vi "UFO.vi"(11 "VI Ref":refnum<vi>) -> ()   [LabVIEW 2019]
doc: "UFO disaster. A UFO will spawn at a random location on the top edge of the screen, then slowly move down the screen destroying any objects in its path."
uses:
  _SubVIs/UFO State Enum.ctl
  _SubVIs/Slave Window Command Message.ctl
  _SubVIs/Slave Window Command.ctl
  _Sound/Music Player Command Message.ctl
  _Sound/Music Player Command.ctl
  _2D/Point.ctl
  <vilib>/Utility/miscctls.llb/LVRectTypeDef.ctl
  <vilib>/numeric/Random Number (Range).vi
  <vilib>/numeric/Random Number (Range) I64.vi
  <vilib>/numeric/sub_Random U32.vi
  _Window/Window.lvlib
  _Sound/Sound.lvlib
  _2D/2D.lvlib
panel:
  out "Attack":u16(ring)
  out "UFO":u16(ring)
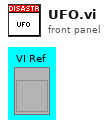
[diagram p1: front panel]
types:
  T1 = enum32{"Invalid", "Standard", "Closed", "Hidden", "Minimized", "Maximized"}
  T2 = typedef "LVRectTypeDef.ctl" = cluster{"Left":i16, "Top":i16, "Right":i16, "Bottom":i16}
  T3 = typedef "2D.lvlib/Point.ctl" = cluster{"X":i16, "Y":i16}
  T4 = typedef "UFO State Enum.ctl" = enum16{"Init", "Init Window", "Play Music", "Fade In Window", "Update Time", "Update Window Position", "Check Window Over BD", "Object Collision Detection", "Update Graphic", "Fade Out Window", "Close Window"}
  T5 = typedef "Sound.lvlib/Music Player Command Message.ctl" = cluster{"Command":T6, "Data":variant}
  T6 = typedef "Sound.lvlib/Music Player Command.ctl" = enum16{"Enable", "Play", "Play Random", "Stop", "Shutdown"}
  T7 = typedef "Slave Window Command Message.ctl" = cluster{"Command":T8, "Data":variant}
  T8 = typedef "Slave Window Command.ctl" = enum16{"Open", "Set Bounds", "Set Opacity", "Close", "Frame"}
  T9 = cluster{"BDWin.NativeWindow":u64, "vi reference":refnum<vi>}[]
  T10 = typedef "LVPointTypeDef.ctl" = cluster{"Horizontal":i16, "Vertical":i16}
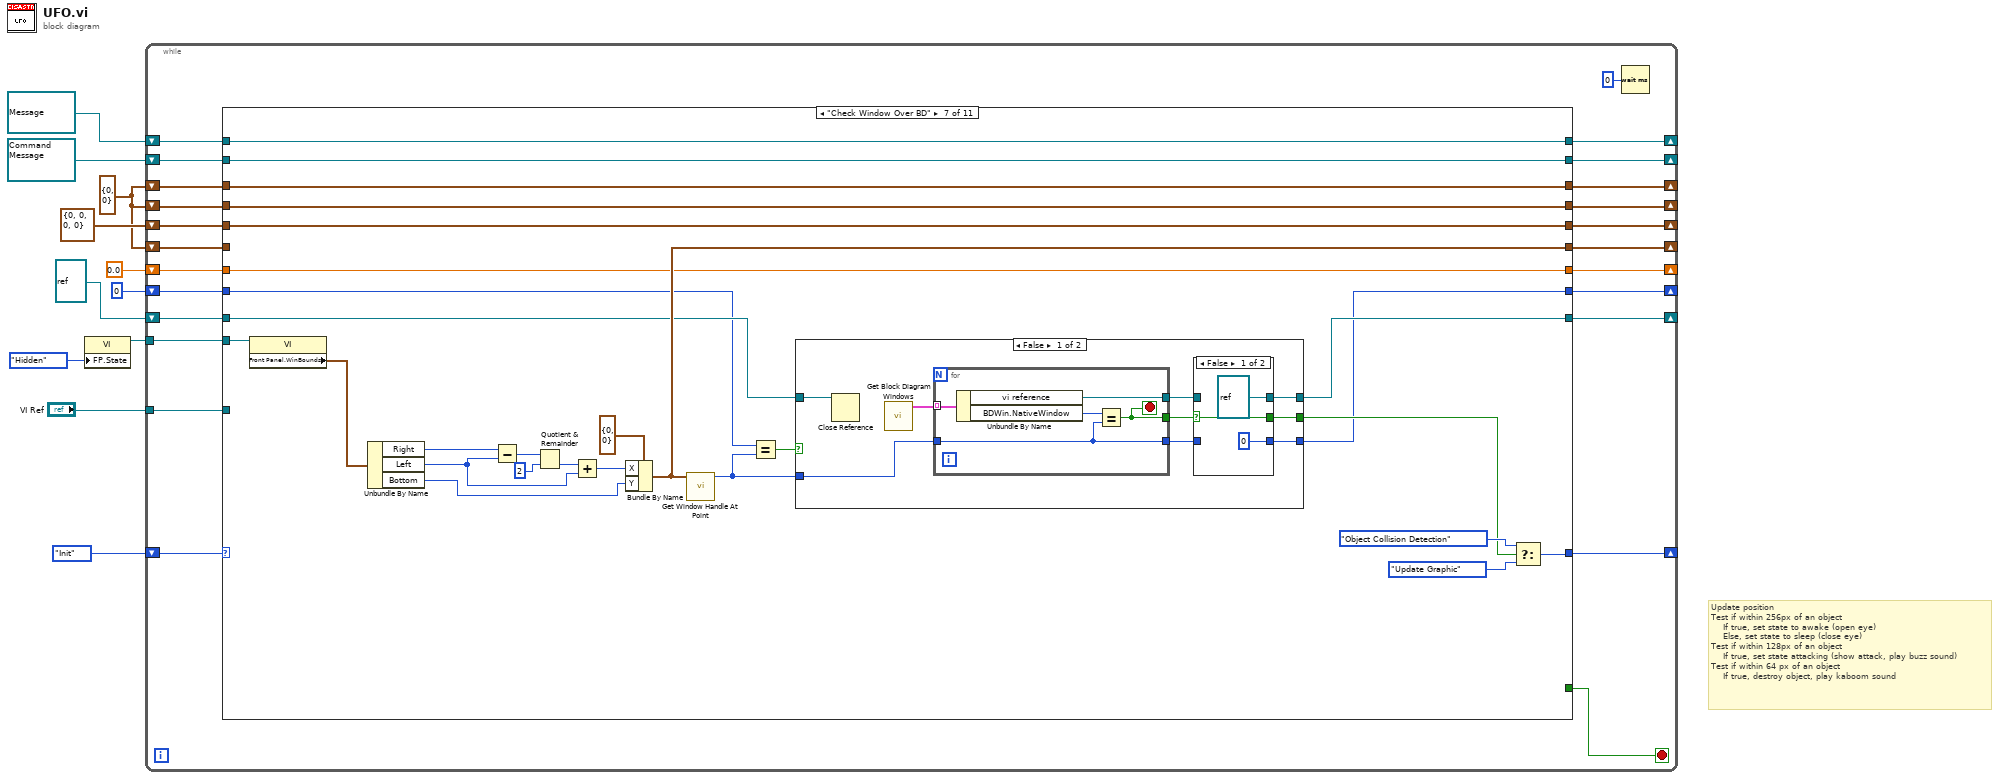
[diagram p0: block diagram]
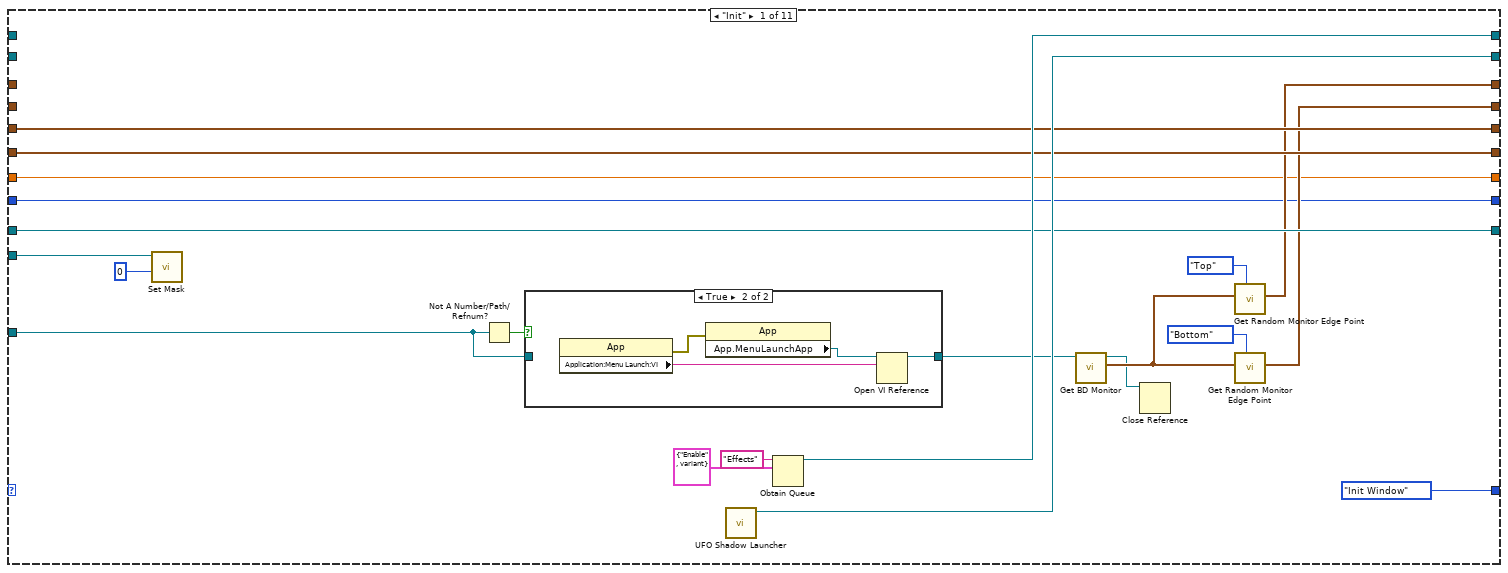
[diagram p2: hidden frame]
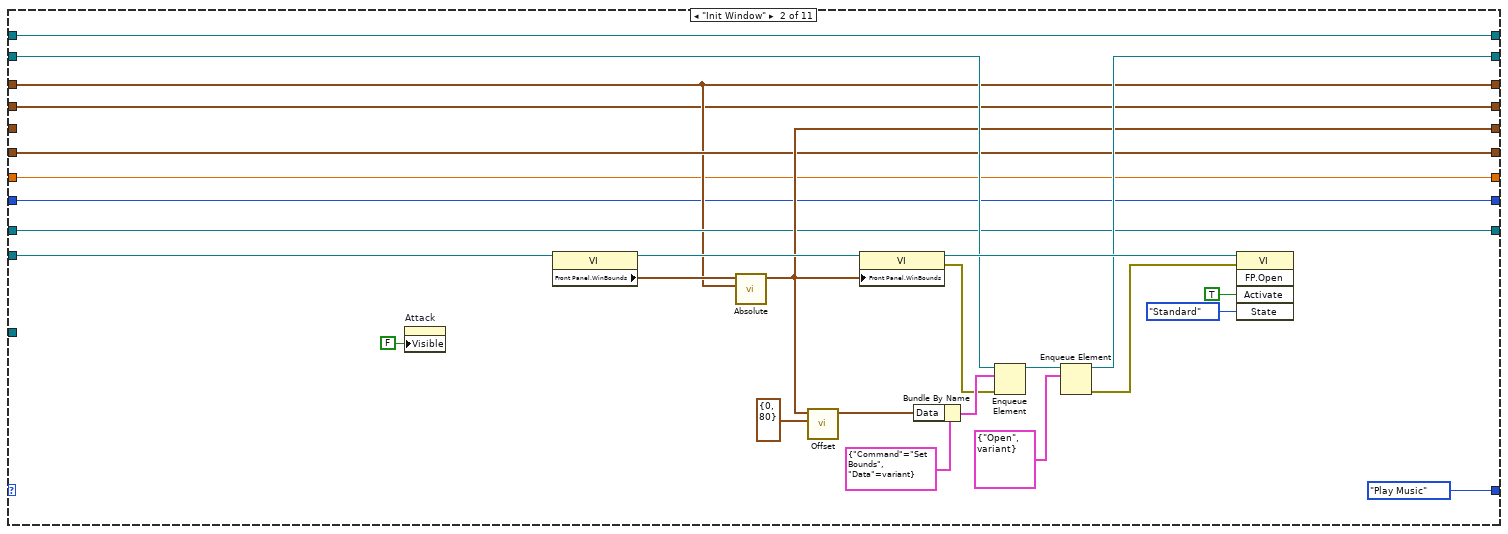
[diagram p4: hidden frame]
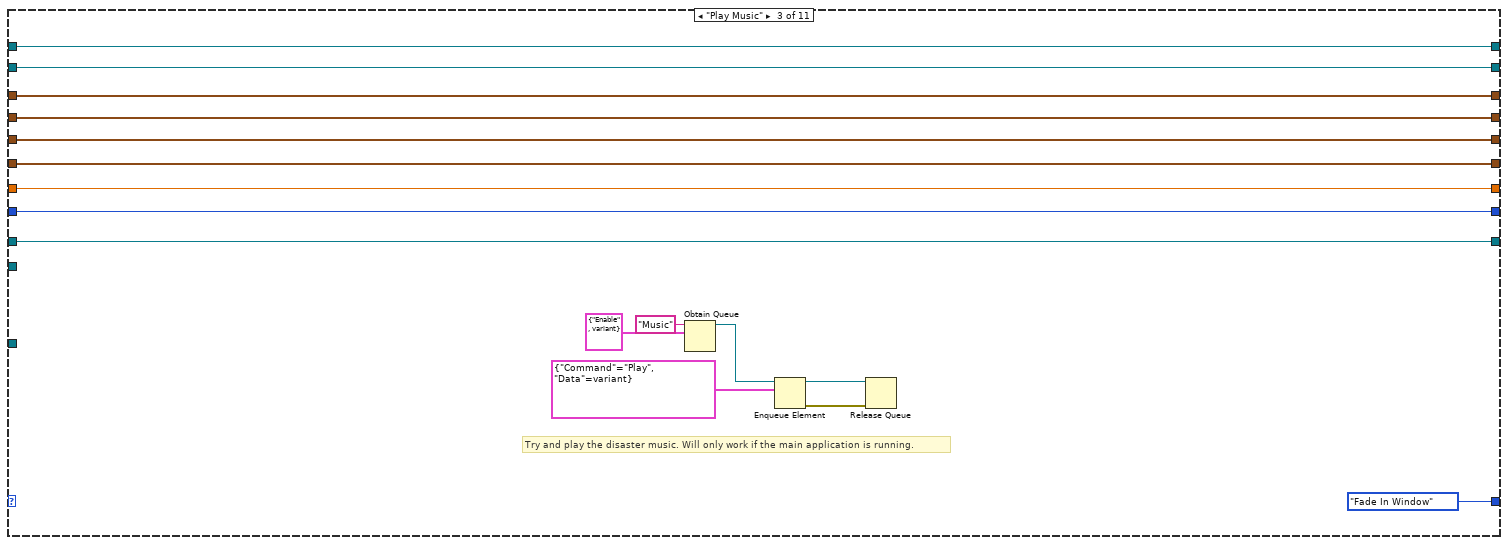
[diagram p5: hidden frame]
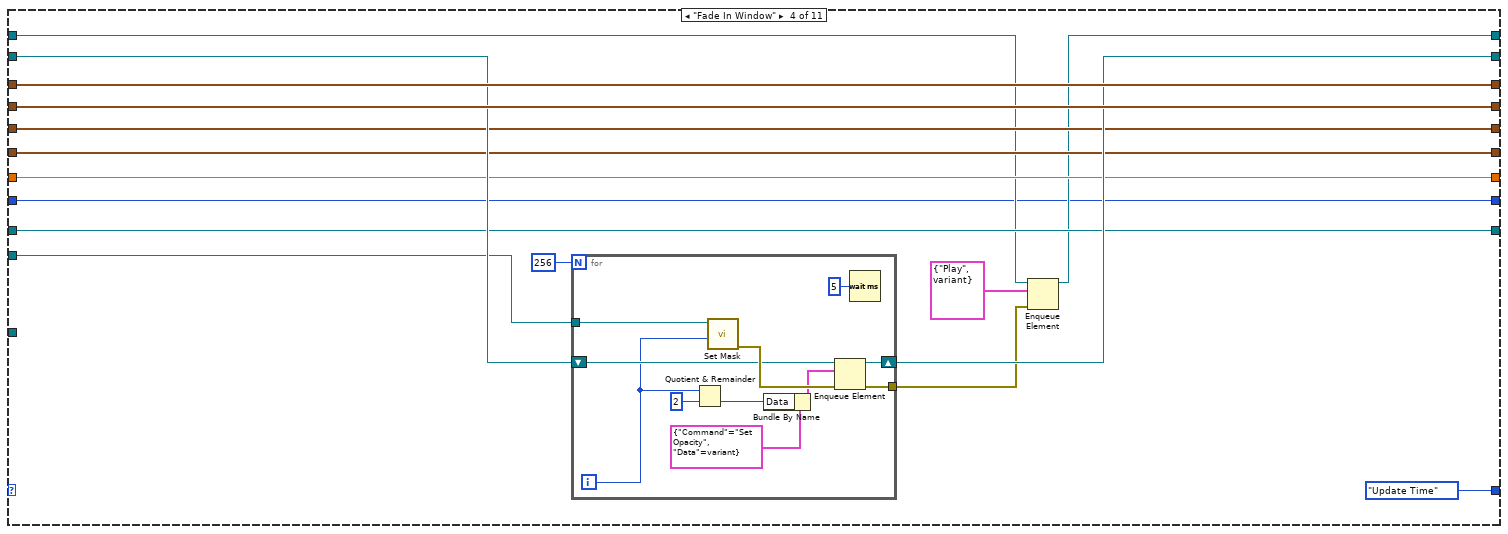
[diagram p6: hidden frame]
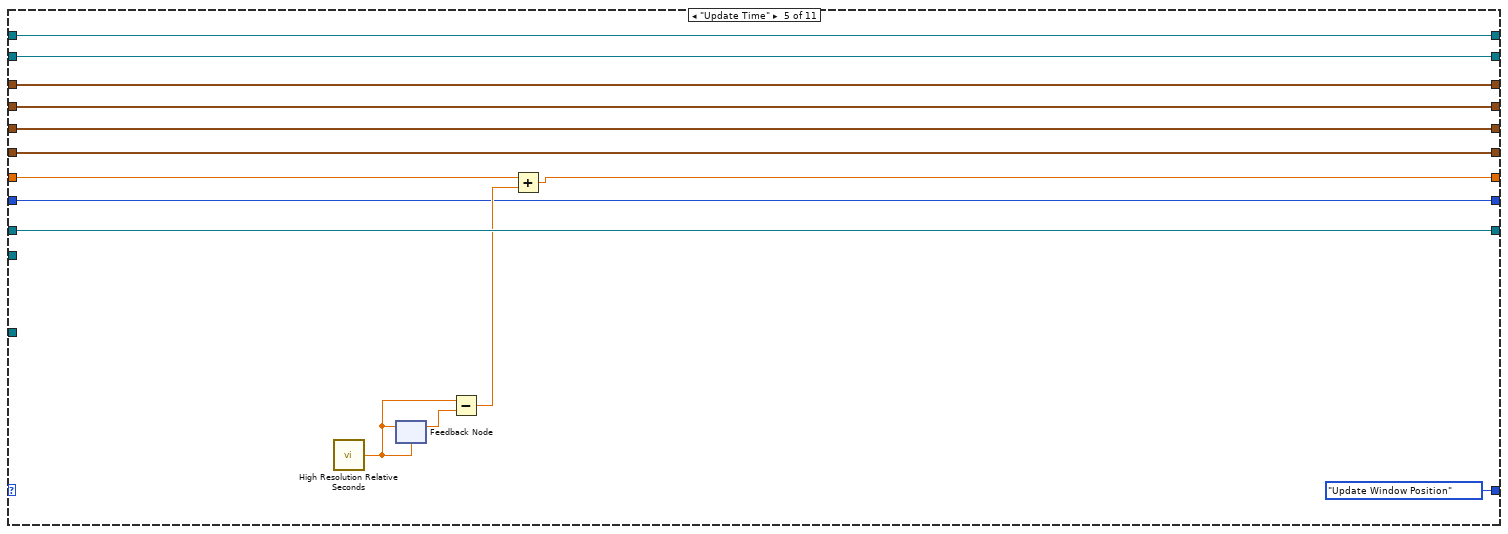
[diagram p7: hidden frame]
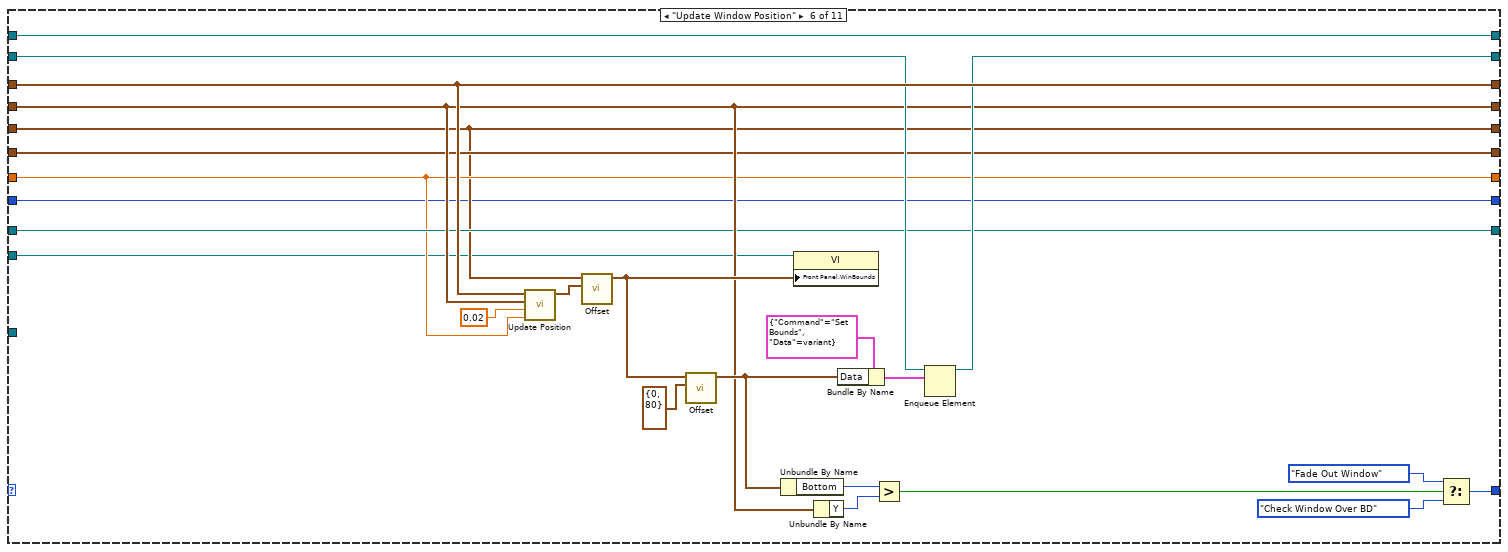
[diagram p8: hidden frame]
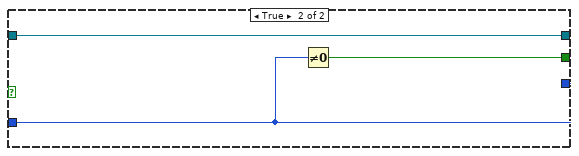
[diagram p10: hidden frame]
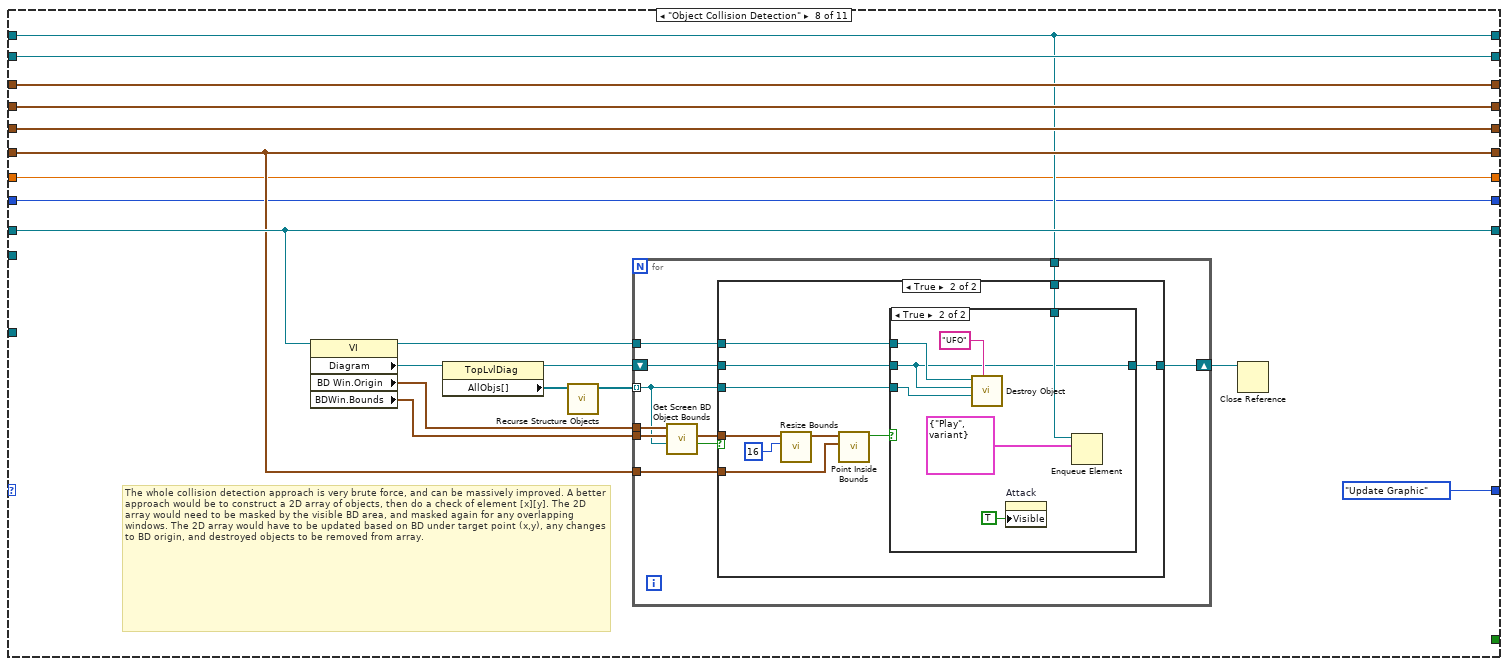
[diagram p11: hidden frame]
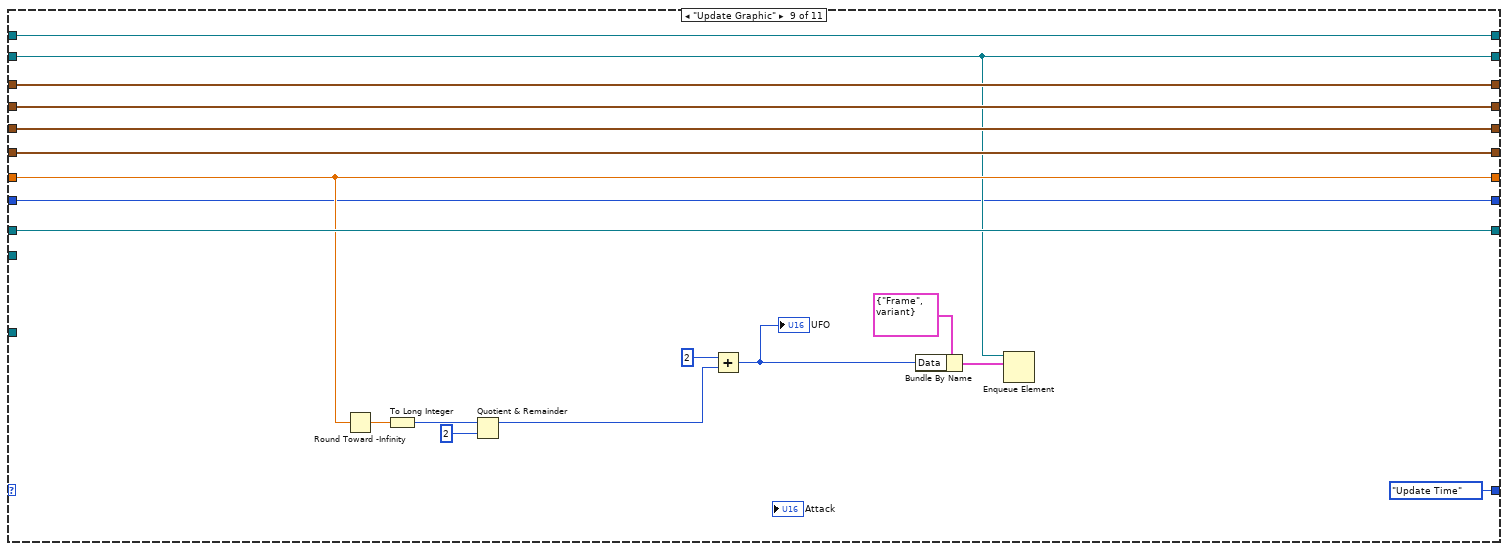
[diagram p14: hidden frame]
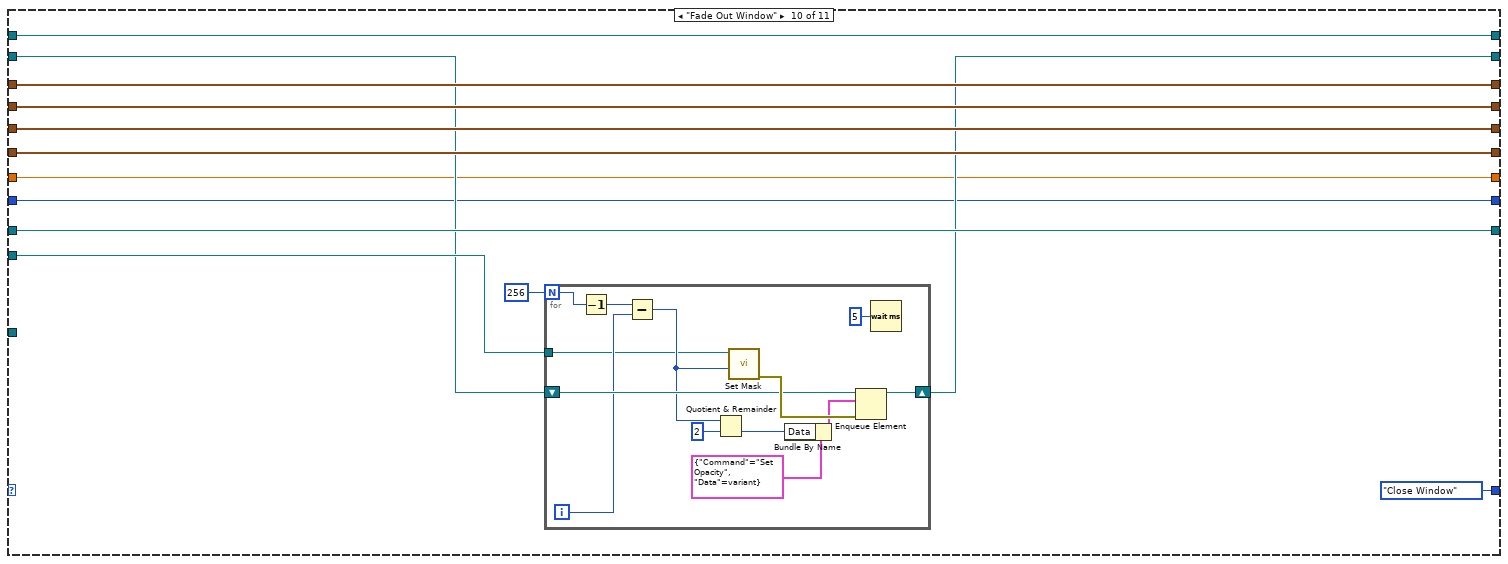
[diagram p15: hidden frame]
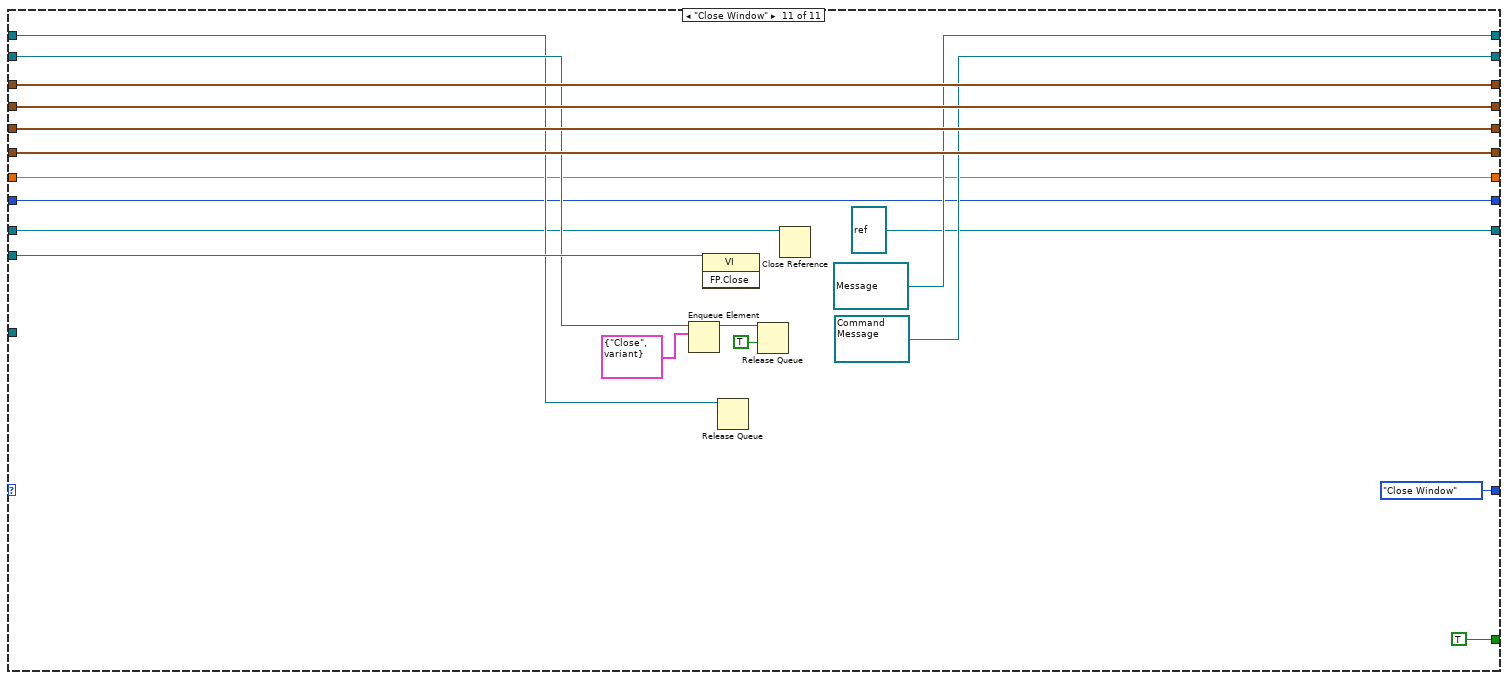
[diagram p16: hidden frame]
diagram:
  w6 = T3 {"X"=0, "Y"=0} ("Point")
  # "Update position\nTest if within 256px of an object\n    If true, set state to awake (open eye)\n    Else, set state to sleep (close eye)\nTest if within 128px of an object\n    If true, set state attacking (show attack, play buzz sound)\nTest if within 64 px of an object\n    If true, destroy object, play kaboom sound"
  n1 = property class="VI"("FP.State"=T1."Hidden" ("Front Panel Window:State")) -> (reference out=w2:refnum<vi>)  [unwired: 2 in, 1 out]
  n2 = while {
    shift-right: [w31] -> _
    shift-left: UFO_State_Enum."Init" -> [w35]
    tunnel: w2 -> [w30]
    shift-right: [w33] -> _
    shift-left: refnum<queue> refnum ("Command Queue") -> [w29]
    shift-right: [w32] -> _
    shift-left: refnum<queue> refnum ("queue out") -> [w28]
    shift-right: [w27] -> _
    shift-left: w6 -> [w25]
    shift-right: [w26] -> _
    shift-left: w6 -> [w24]
    shift-right: [w23] -> _
    shift-left: T2 {"Left"=0, "Top"=0, "Right"=0, "Bottom"=0} ("Bounds Out") -> [w22]
    shift-right: [w21] -> _
    shift-left: refnum<vi> refnum ("vi reference") -> [w18]
    shift-right: [w20] -> _
    shift-left: w6 -> [w19]
    tunnel: "VI Ref" -> [w34]
    shift-right: [w15] -> _
    shift-left: 0.0 -> [w16]
    shift-right: [w13] -> _
    shift-left: 0 ("hWnd") -> [w12]
    stop <- w17 stop-if-true
    n3 = case shown="\"Check Window Over BD\"" w35 {
      tunnel: w34 -> [w54 _ _ _ _ _ _ _ _ _ _]
      tunnel: [w52 w69 w96 w116 w144 w157 w195 w236 w274 w288 refnum<queue> refnum ("Command Queue")] -> w33
      tunnel: [w51 w70 w97 w107 w143 w168 w194 w222 w283 w296 refnum<queue> refnum ("queue out")] -> w32
      tunnel: [UFO_State_Enum."Init Window" UFO_State_Enum."Play Music" UFO_State_Enum."Fade In Window" UFO_State_Enum."Update Time" UFO_State_Enum."Update Window Position" w152 w180 UFO_State_Enum."Update Graphic" UFO_State_Enum."Update Time" UFO_State_Enum."Close Window" UFO_State_Enum."Close Window"] -> w31
      tunnel: w30 -> [w38 w74 _ w110 _ w146 w182 _ _ w289 w320]
      tunnel: w29 -> [_ w72 w96 w115 w144 w156 w195 w236 w274 w287 w319]
      tunnel: w28 -> [_ w70 w97 w106 w143 w168 w194 w222 w283 w296 w318]
      tunnel: [w42 w65 w95 w118 w142 w158 w193 w235 w282 w295 w327] -> w27
      tunnel: [w41 w64 w94 w117 w141 w151 w192 w234 w281 w294 w326] -> w26
      tunnel: w25 -> [_ w65 w95 w118 w142 w158 w193 w235 w282 w295 w327]
      tunnel: w24 -> [_ w64 w94 w117 w141 w151 w192 w234 w281 w294 w326]
      tunnel: [w49 w68 w92 w113 w140 w147 w191 w233 w280 w293 w325] -> w23
      tunnel: w22 -> [w49 _ w92 w113 w140 w147 w191 w233 w280 w293 w325]
      tunnel: [w47 w66 w90 w111 w139 w149 w174 w227 w279 w292 refnum<vi> refnum ("vi reference")] -> w21
      tunnel: [w48 w67 w91 w112 w138 w150 w177 w226 w278 w291 w324] -> w20
      tunnel: w19 -> [w48 w67 w91 w112 w138 w150 _ w226 w278 w291 w324]
      tunnel: w18 -> [w47 w66 w90 w111 w139 w149 w173 w227 w279 w292 w311]
      tunnel: [_ _ _ _ _ _ _ _ _ _ TRUE] -> w17
      tunnel: w16 -> [w40 w63 w89 w109 w135 w148 w176 w221 w275 w285 w313]
      tunnel: [w40 w63 w89 w109 w132 w148 w176 w221 w275 w285 w313] -> w15
      tunnel: [w37 w62 w88 w104 w131 w145 w172 w220 w266 w284 w312] -> w13
      tunnel: w12 -> [w37 w62 w88 w104 w131 w145 w171 w220 w266 w284 w312]
      frame "Init" {
        n4 = call "Set Mask.vi"("Alpha (255)"=0, "VI Ref In"=w38) -> ()  [unwired: 8 in, 2 out]
        n5 = Not A Number/Path/Refnum?(number/path/refnum=w54) -> (NaN/Path/Refnum?=w53:bool)
        n6 = case shown="True" w53 {
          tunnel: w54 -> [w57 _]
          tunnel: [w57 w60] -> w43
          frame False {
          }
          frame True {
            n7 = property class="App"() -> (error out=w59:errorcluster, "Application:Menu Launch:VI"=w61:string)  [unwired: 2 in, 1 out]
            n8 = property class="App"(error in=w59) -> ("App.MenuLaunchApp"=w58:refnum<vi>)  [unwired: 1 in, 2 out]
            n9 = Open VI Reference(application reference (local)=w58, vi path=w61) -> (vi reference=w60:refnum<vi>)  [unwired: 4 in, 1 out]
          }
        }
        n10 = call "UFO Shadow Launcher.vi"() -> ("Command Queue"=w52:refnum<queue>)  [unwired: 10 in, 1 out]
        n11 = Obtain Queue(name (unnamed)="Effects", element data type=T5 {"Command"=enum."Enable", "Data"=variant} ("Message")) -> (queue out=w51:refnum<queue>)  [unwired: 3 in, 2 out]
        n12 = call "Get BD Monitor.vi"("VI Ref In"=w43) -> ("Monitor Bounds"=w46:T2, "VI Ref Out"=w36:refnum<vi>)  [unwired: 8 in, 1 out]
        n13 = Close Reference(reference=w36) -> ()  [unwired: 1 in, 1 out]
        n14 = call "Get Random Monitor Edge Point.vi"("Edge"=enum16{"Left", "Top", "Right", "Bottom"}."Top", "Monitor Bounds"=w46) -> ("Point"=w42:T3)  [unwired: 9 in]
        n15 = call "Get Random Monitor Edge Point.vi"("Edge"=enum16{"Left", "Top", "Right", "Bottom"}."Bottom", "Monitor Bounds"=w46) -> ("Point"=w41:T3)  [unwired: 9 in]
      }
      frame "Init Window" {
        n16 = property on="Attack" class="Ring (strict)"("Visible"=FALSE) -> ()  [unwired: 2 in, 2 out]
        n17 = property class="VI"(reference=w74) -> (reference out=w77:refnum<vi>, "Front Panel.WinBounds"=w84:T2)  [unwired: 1 in, 1 out]
        n18 = call "Absolute.vi"("Point"=w65, "Bounds In"=w84) -> ("Bounds Out"=w68:T2)  [unwired: 9 in]
        n19 = call "Offset.vi"("Point"=T3 {"X"=0, "Y"=80}, "Bounds In"=w68) -> ("Bounds Out"=w85:T2)  [unwired: 9 in]
        n20 = property class="VI"(reference=w77, "Front Panel.WinBounds"=w68) -> (reference out=w78:refnum<vi>, error out=w73:errorcluster)  [unwired: 1 in]
        n21 = Bundle By Name(cluster=T7 {"Command"=enum."Set Bounds", "Data"=variant} ("Command Message"), "Data"=w85) -> (w80:T7)
        n22 = Enqueue Element(queue=w72, element=w80, error in (no error)=w73) -> (queue out=w82:refnum<queue>)  [unwired: 1 in, 2 out]
        n23 = Enqueue Element(queue=w82, element=T7 {"Command"=enum."Open", "Data"=variant(bool TRUE)} ("Command Message")) -> (queue out=w69:refnum<queue>, error out=w83:errorcluster)  [unwired: 2 in, 1 out]
        n24 = invoke class="VI" method="FP.Open"(reference=w78, error in=w83, "Activate"=TRUE ("Activate?"), "State"=T1."Standard") -> ()  [unwired: 1 in, 5 out]
      }
      frame "Play Music" {
        # "Try and play the disaster music. Will only work if the main application is running."
        n25 = Obtain Queue(name (unnamed)="Music", element data type=T5 {"Command"=enum."Enable", "Data"=variant} ("Message")) -> (queue out=w100:refnum<queue>)  [unwired: 3 in, 2 out]
        n26 = Enqueue Element(queue=w100, element=T5 {"Command"=enum."Play", "Data"=variant(string "Disasters\\Disaster Decision")}) -> (queue out=w99:refnum<queue>, error out=w98:errorcluster)  [unwired: 2 in, 1 out]
        n27 = Release Queue(queue=w99, error in (no error)=w98) -> ()  [unwired: 1 in, 3 out]
      }
      frame "Fade In Window" {
        n28 = for {
          N: 256 -> [_]
          shift-right: [w128] -> w116
          shift-left: w115 -> [w127]
          tunnel: w110 -> [w121]
          tunnel: [w120] -> w105
          i -> [w126]
          n29 = Quotient & Remainder(x=w126, y=2) -> (floor(x/y)=w123:i32)  [unwired: 1 out]
          n30 = call "Set Mask.vi"("Alpha (255)"=w126, "VI Ref In"=w121) -> ("error out"=w129:errorcluster)  [unwired: 8 in, 1 out]
          n31 = Bundle By Name(cluster=T7 {"Command"=enum."Set Opacity", "Data"=variant} ("Command Message"), "Data"=w123) -> (w122:T7)
          n32 = Enqueue Element(queue=w127, element=w122, error in (no error)=w129) -> (queue out=w128:refnum<queue>, error out=w120:errorcluster)  [unwired: 1 in, 1 out]
          n33 = Wait (ms)(milliseconds to wait=u32 5) -> ()  [unwired: 1 out]
        }
        n34 = Enqueue Element(queue=w106, element=T5 {"Command"=enum."Play", "Data"=variant(string "siren")}, error in (no error)=w105) -> (queue out=w107:refnum<queue>)  [unwired: 1 in, 2 out]
      }
      frame "Update Time" {
        n35 = call <vilib>:"High Resolution Relative Seconds.vi"() -> ("relative seconds"=w133:dbl)
        n36 = feedback-in #1(w133) -> ()
        n37 = feedback #1(w133) -> (w137:dbl)
        n38 = Subtract(x=w133, y=w137) -> (x-y=w134:dbl)
        n39 = Add(x=w135, y=w134) -> (x+y=w132:dbl)
      }
      frame "Update Window Position" {
        n40 = call "Update Position.vi"("Time"=w148, "Speed"=0.02 ("Speed (px/sec)"), "End Pos"=w151, "Start Pos"=w158) -> ("Current Pos"=w162:T3)  [unwired: 7 in]
        n41 = call "Offset.vi"("Point"=w162, "Bounds In"=w147) -> ("Bounds Out"=w160:T2)  [unwired: 9 in]
        n42 = call "Offset.vi"("Point"=T3 {"X"=0, "Y"=80}, "Bounds In"=w160) -> ("Bounds Out"=w159:T2)  [unwired: 9 in]
        n43 = Unbundle By Name(w159) -> ("Bottom"=w165:i16)
        n44 = property class="VI"(reference=w146, "Front Panel.WinBounds"=w160) -> ()  [unwired: 1 in, 2 out]
        n45 = Unbundle By Name(w151) -> ("Y"=w164:i16)
        n46 = Bundle By Name(cluster=T7 {"Command"=enum."Set Bounds", "Data"=variant} ("Command Message"), "Data"=w159) -> (w166:T7)
        n47 = Greater?(x=w165, y=w164) -> (0:w155:bool)
        n48 = Enqueue Element(queue=w156, element=w166) -> (queue out=w157:refnum<queue>)  [unwired: 2 in, 2 out]
        n49 = Select(t=UFO_State_Enum."Fade Out Window", s=w155, f=UFO_State_Enum."Check Window Over BD") -> (s? t:f=w152:T4)
      }
      frame "Check Window Over BD" {
        n50 = property class="VI"(reference=w182) -> ("Front Panel.WinBounds"=w181:T2)  [unwired: 1 in, 2 out]
        n51 = Unbundle By Name(w181) -> ("Right"=w190:i16, "Left"=w186:i16, "Bottom"=w183:i16)
        n52 = Subtract(x=w190, y=w186) -> (x-y=w189:i16)
        n53 = Quotient & Remainder(x=w189, y=i16 2) -> (floor(x/y)=w187:i16)  [unwired: 1 out]
        n54 = Add(x=w187, y=w186) -> (x+y=w184:i16)
        n55 = Bundle By Name(cluster=T3 {"X"=0, "Y"=0} ("Point"), "X"=w184, "Y"=w183) -> (w177:T3)
        n56 = call "Get Window Handle At Point.vi"("Point"=w177) -> ("hWnd"=w170:i32)  [unwired: 9 in, 1 out]
        n57 = Equal?(x=w171, y=w170) -> (x = y?=w169:bool)
        n58 = case shown="False" w169 {
          tunnel: w170 -> [w203 w216]
          tunnel: [w200 w217] -> w175
          tunnel: [w197 w218] -> w174
          tunnel: [w196 w216] -> w172
          tunnel: w173 -> [w202 w218]
          frame False {
            n59 = Close Reference(reference=w202) -> ()  [unwired: 1 in, 1 out]
            n60 = call "Get Block Diagram Windows.vi"() -> ("VIs With Open BDs"=w204:T9)  [unwired: 11 in]
            n61 = for {
              tunnel: w204 -> [w215] mode=indexing
              tunnel: [w214] -> w198
              tunnel: [w213] -> w201
              tunnel: w203 -> [w211]
              tunnel: [w211] -> w199
              stop <- w213 stop-if-true
              n62 = Unbundle By Name(w215) -> ("vi reference"=w214:refnum<vi>, "BDWin.NativeWindow"=w212:u64)
              n63 = Equal?(x=w212, y=w211) -> (x = y?=w213:bool)
            }
            n64 = case shown="False" w201 {
              selector: w201 -> [w207 w210]
              tunnel: [w207 w210] -> w200
              tunnel: w199 -> [_ w208]
              tunnel: w198 -> [_ w209]
              tunnel: [refnum<vi> refnum ("vi reference") w209] -> w197
              tunnel: [0 ("hWnd") w208] -> w196
              frame False {
              }
              frame True {
              }
            }
          }
          frame True {
            n65 = Not Equal To 0?(x=w216) -> (x != 0?=w217:bool)
          }
        }
        n66 = Select(t=UFO_State_Enum."Object Collision Detection", s=w175, f=UFO_State_Enum."Update Graphic") -> (s? t:f=w180:T4)
      }
      frame "Object Collision Detection" {
        # "The whole collision detection approach is very brute force, and can be massively improved. A better approach would be to construct a 2D array of objects, then do a check of element [x][y]. The 2D array would need to be masked by the visible BD area, and masked again for any overlapping windows. The 2D array would have to be updated based on BD under target point (x,y), any changes to BD origin, and destroyed objects to be removed from array."
        n67 = property class="VI"(reference=w227) -> (reference out=w229:refnum<vi>, "Diagram"=w231:refnum<vi>, "BD Win.Origin"=w225:T10, "BDWin.Bounds"=w224:T2)  [unwired: 1 in, 1 out]
        n68 = property class="TopLvlDiag"(reference=w231) -> (reference out=w228:refnum<vi>, "AllObjs[]"=w232:refnum<vi>[])  [unwired: 1 in, 1 out]
        n69 = call "Recurse Structure Objects.vi"("Objects In"=w232) -> ("Objects Out"=w230:refnum<vi>[])  [unwired: 10 in]
        n70 = for {
          tunnel: w225 -> [w246]
          tunnel: w224 -> [w245]
          tunnel: w230 -> [w240] mode=indexing
          tunnel: w226 -> [w242]
          tunnel: w229 -> [w241]
          tunnel: w222 -> [w238]
          shift-right: [w237] -> w219
          shift-left: w228 -> [w239]
          n71 = call "Get Screen BD Object Bounds.vi"("Object Reference"=w240, "BD Window Bounds"=w245, "BD Origin"=w246) -> ("Object Visible?"=w244:bool, "Screen Object Bounds"=w243:T2)  [unwired: 6 in, 1 out]
          n72 = case shown="True" w244 {
            tunnel: w243 -> [_ w257]
            tunnel: w242 -> [_ w254]
            tunnel: w241 -> [_ w250]
            tunnel: w240 -> [_ w252]
            tunnel: w239 -> [w247 w251]
            tunnel: w238 -> [_ w249]
            tunnel: [w247 w248] -> w237
            frame False {
            }
            frame True {
              n73 = call "Resize Bounds.vi"("Resize Amount"=i16 16, "Bounds In"=w257) -> ("Bounds Out"=w255:T2)  [unwired: 9 in]
              n74 = call "Point Inside Bounds.vi"("Point"=w254, "Bounds"=w255) -> ("Inside?"=w253:bool)  [unwired: 9 in]
              n75 = case shown="True" w253 {
                tunnel: w252 -> [_ w264]
                tunnel: w251 -> [w258 w259]
                tunnel: w250 -> [_ w263]
                tunnel: w249 -> [_ w261]
                tunnel: [w258 w259] -> w248
                frame False {
                }
                frame True {
                  n76 = call "Destroy Object.vi"("Undo Text"="UFO", "Object Ref"=w264, "BD Ref"=w259, "VI Ref"=w263) -> ()  [unwired: 7 in, 1 out]
                  n77 = property on="Attack" class="Ring (strict)"("Visible"=TRUE) -> ()  [unwired: 2 in, 2 out]
                  n78 = Enqueue Element(queue=w261, element=T5 {"Command"=enum."Play", "Data"=variant(string "kaboom")}) -> ()  [unwired: 2 in, 3 out]
                }
              }
            }
          }
        }
        n79 = Close Reference(reference=w219) -> ()  [unwired: 1 in, 1 out]
      }
      frame "Update Graphic" {
        n80 = Round Toward -Infinity(1:w275) -> (0:w272:dbl)
        n81 = To Long Integer(number=w272) -> (32bit integer=w273:i32)
        n82 = Quotient & Remainder(x=w273, y=2) -> (x-y*floor(x/y)=w267:i32)  [unwired: 1 out]
        n83 = Add(x=i16 2, y=w267) -> (x+y=w268:i32)
        "UFO" <- w268
        n84 = Bundle By Name(cluster=T7 {"Command"=enum."Frame", "Data"=variant} ("Command Message"), "Data"=w268) -> (w270:T7)
        n85 = Enqueue Element(queue=w274, element=w270) -> ()  [unwired: 2 in, 3 out]
      }
      frame "Fade Out Window" {
        n86 = for {
          N: 256 -> [w301]
          shift-right: [w307] -> w288
          shift-left: w287 -> [w306]
          tunnel: w289 -> [w297]
          i -> [w299]
          n87 = Decrement(x=w301) -> (x-1=w300:i32)
          n88 = Subtract(x=w300, y=w299) -> (x-y=w298:i32)
          n89 = Quotient & Remainder(x=w298, y=2) -> (floor(x/y)=w303:i32)  [unwired: 1 out]
          n90 = call "Set Mask.vi"("Alpha (255)"=w298, "VI Ref In"=w297) -> ("error out"=w308:errorcluster)  [unwired: 8 in, 1 out]
          n91 = Bundle By Name(cluster=T7 {"Command"=enum."Set Opacity", "Data"=variant} ("Command Message"), "Data"=w303) -> (w302:T7)
          n92 = Enqueue Element(queue=w306, element=w302, error in (no error)=w308) -> (queue out=w307:refnum<queue>)  [unwired: 1 in, 2 out]
          n93 = Wait (ms)(milliseconds to wait=u32 5) -> ()  [unwired: 1 out]
        }
      }
      frame "Close Window" {
        n94 = Enqueue Element(queue=w319, element=T7 {"Command"=enum."Close", "Data"=variant}) -> (queue out=w322:refnum<queue>)  [unwired: 2 in, 2 out]
        n95 = invoke class="VI" method="FP.Close"(reference=w320) -> ()  [unwired: 2 in, 3 out]
        n96 = Release Queue(queue=w318) -> ()  [unwired: 2 in, 3 out]
        n97 = Release Queue(queue=w322, force destroy? (F)=TRUE) -> ()  [unwired: 1 in, 3 out]
        n98 = Close Reference(reference=w311) -> ()  [unwired: 1 in, 1 out]
      }
    }
    n99 = Wait (ms)(milliseconds to wait=u32 0) -> ()  [unwired: 1 out]
  }
